vi "2GaussianFit.vi"(0 "x":dbl[](array[numeric]), 1 "Histogram(x)":i32[](array[numeric])) -> (2 "Sum":cluster{"X":dbl[], dbl[]}, 3 "Peak 2":dbl[][](array[numeric]), 4 "Peak 1":dbl[][](array[numeric]))   [LabVIEW 2009]
uses:
  <vilib>/gmath/NI_Gmath.lvlib
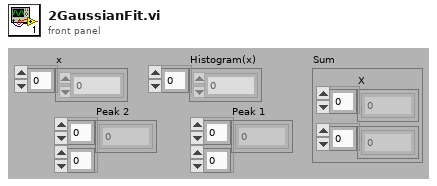
[diagram p1: front panel]
types:
  T1 = cluster{"Array[0]":dbl, "Array[1]":dbl, "Array[2]":dbl, "Array[3]":dbl, "Array[4]":dbl, "Array[5]":dbl, "Array[6]":dbl, "Array[7]":dbl, "Array[8]":dbl}
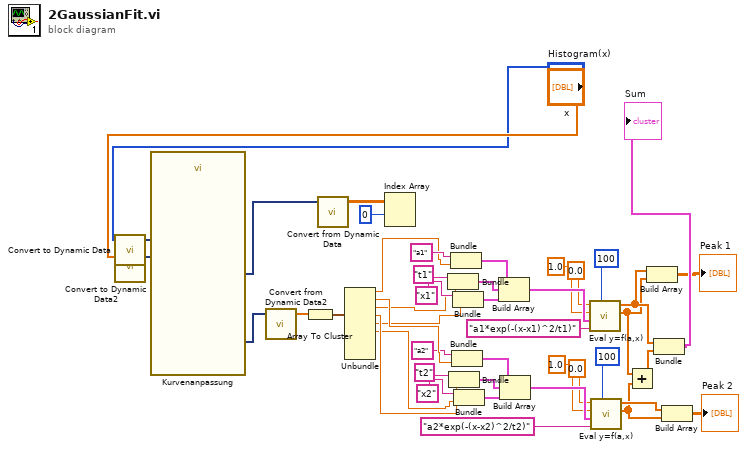
[diagram p0: block diagram]
diagram:
  n1 = call "Convert to Dynamic Data"("Array"="Histogram(x)") -> ("Dynamic Data Type"=w10:dynamicdata)  [unwired: 3 in]
  n2 = call "Convert to Dynamic Data2"("Array"="x") -> ("Dynamic Data Type"=w11:dynamicdata)  [unwired: 3 in]
  n3 = call "Kurvenanpassung"("Locations"=w11, "Signals"=w10) -> ("best fit"=w7:dynamicdata, "non-linear coefficients"=w12:dynamicdata)  [unwired: 5 in, 3 out]
  n4 = call "Convert from Dynamic Data2"("Dynamic Data Type"=w12) -> ("Array"=w15:dbl[])  [unwired: 3 in]
  n5 = Array To Cluster(array=w15) -> (cluster=w16:T1)
  n6 = call "Convert from Dynamic Data"("Dynamic Data Type"=w7) -> ("Array"=w9:dbl[][])  [unwired: 3 in]
  n7 = Unbundle(w16) -> ("Array[0]"=w25:dbl, "Array[1]"=w44:dbl, "Array[2]"=w26:dbl, "Array[3]"=w43:dbl, "Array[4]"=w27:dbl, "Array[5]"=w42:dbl)  [unwired: 3 out]
  n8 = Index Array(array=w9, index (row)=0) -> ()  [unwired: 1 in, 1 out]
  n9 = Bundle("t1", "Array[2]"=w26) -> (w23:cluster{string, "Array[2]":dbl})  [unwired: 1 in]
  n10 = Bundle("t2", "Array[3]"=w43) -> (w37:cluster{string, "Array[3]":dbl})  [unwired: 1 in]
  n11 = Bundle("a1", "Array[0]"=w25) -> (w24:cluster{string, "Array[0]":dbl})  [unwired: 1 in]
  n12 = Bundle("a2", "Array[1]"=w44) -> (w38:cluster{string, "Array[1]":dbl})  [unwired: 1 in]
  n13 = Bundle("x1", "Array[4]"=w27) -> (w22:cluster{string, "Array[4]":dbl})  [unwired: 1 in]
  n14 = Bundle("x2", "Array[5]"=w42) -> (w36:cluster{string, "Array[5]":dbl})  [unwired: 1 in]
  n15 = Build Array(w24, w23, w22) -> (w21:cluster{string, "Array[4]":dbl}[])
  n16 = Build Array(w38, w37, w36) -> (w35:cluster{string, "Array[5]":dbl}[])
  n17 = call <vilib>:"Eval y=f(a,x).vi"("number of points"=u32 100, "formula"="a1*exp(-(x-x1)^2/t1)", "Parameters"=w21, "end"=1.0, "start"=0.0) -> ("Y"=w3:dbl[], "X"=w4:dbl[])  [unwired: 2 out]
  n18 = call <vilib>:"Eval y=f(a,x).vi"("number of points"=u32 100, "formula"="a2*exp(-(x-x2)^2/t2)", "Parameters"=w35, "end"=1.0, "start"=0.0) -> ("Y"=w5:dbl[], "X"=w6:dbl[])  [unwired: 2 out]
  n19 = Add(x=w3, y=w5) -> (x+y=w45:dbl[])
  n20 = Build Array(w4, w3) -> (→"Peak 1":dbl[][])
  n21 = Bundle("X"=w4, w45) -> (→"Sum":cluster{"X":dbl[], dbl[]})  [unwired: 1 in]
  n22 = Build Array(w6, w5) -> (→"Peak 2":dbl[][])
